vi "Coincident edges (indexed) test.vi"(1 "Existing edges (indexed)":T1[](array[typedef]), 2 "Candidate edge (indexed)":T1={"V0"=[], "V1"=[], "i0"=-1, "i1"=-1}) -> (0 "Edge already exists":bool)   [LabVIEW 2014]
uses:
  Typedefs/Edge, indexed.ctl
panel:
  # "PN 29/03/2015"
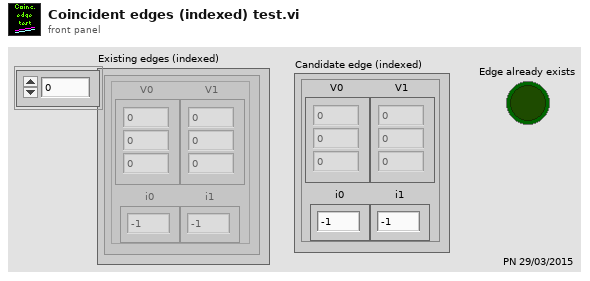
[diagram p1: front panel]
types:
  T1 = typedef "Edge, indexed.ctl" = cluster{"V0":sgl[], "V1":sgl[], "i0":i32, "i1":i32}
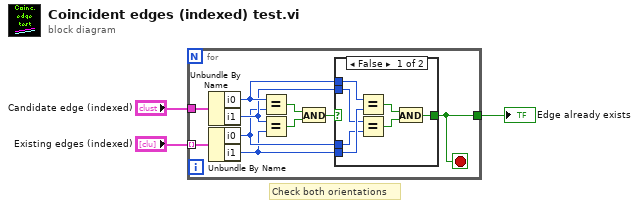
[diagram p0: block diagram]
diagram:
  # "Check both orientations"
  n1 = for {
    tunnel: "Existing edges (indexed)" -> [w13] mode=indexing
    tunnel: "Candidate edge (indexed)" -> [w12]
    tunnel: [w8] -> w2
    stop <- w8 stop-if-true
    n2 = Unbundle By Name(w12) -> ("i0"=w7:i32, "i1"=w6:i32)
    n3 = Unbundle By Name(w13) -> ("i0"=w5:i32, "i1"=w4:i32)
    n4 = Equal?(x=w7, y=w5) -> (x = y?=w11:bool)
    n5 = Equal?(x=w6, y=w4) -> (x = y?=w10:bool)
    n6 = And(x=w11, y=w10) -> (x .and. y?=w9:bool)
    n7 = case shown="False" w9 {
      selector: w9 -> [_ w21]
      tunnel: [w18 w21] -> w8
      tunnel: w7 -> [w17 _]
      tunnel: w6 -> [w15 _]
      tunnel: w5 -> [w14 _]
      tunnel: w4 -> [w16 _]
      frame False {
        n8 = Equal?(x=w17, y=w16) -> (x = y?=w19:bool)
        n9 = Equal?(x=w15, y=w14) -> (x = y?=w20:bool)
        n10 = And(x=w19, y=w20) -> (x .and. y?=w18:bool)
      }
      frame True {
      }
    }
  }
  "Edge already exists" <- w2
